vi "FGV test.vi"() -> ()   [LabVIEW 2023]
uses:
  CONTROLS/fgv-status.ctl
panel:
  in  "fgv-status 2":T1
  out "Preis Output 2":dbl
  out "error out":errorcluster
  in  "Preis Input":dbl format="%#_13g"
  in  "error in":errorcluster
  in  "fgv-status":T1
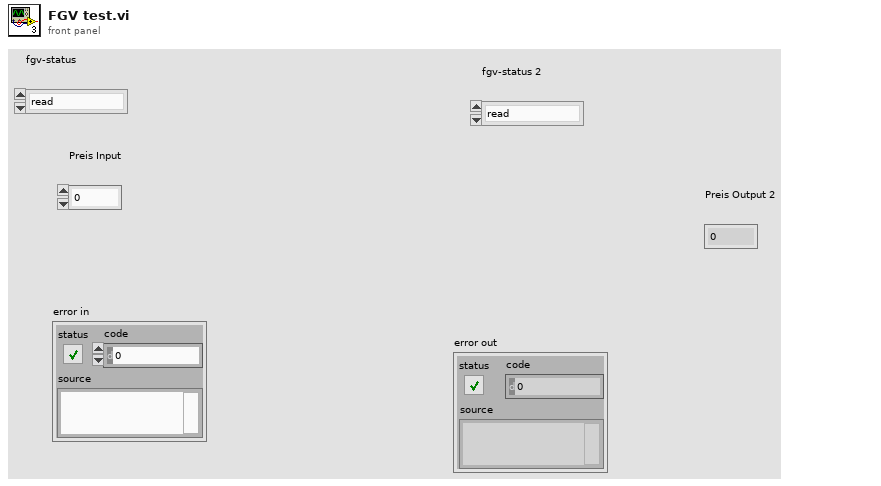
[diagram p1: front panel]
types:
  T1 = typedef "fgv-status.ctl" = enum16{"read", "write"}
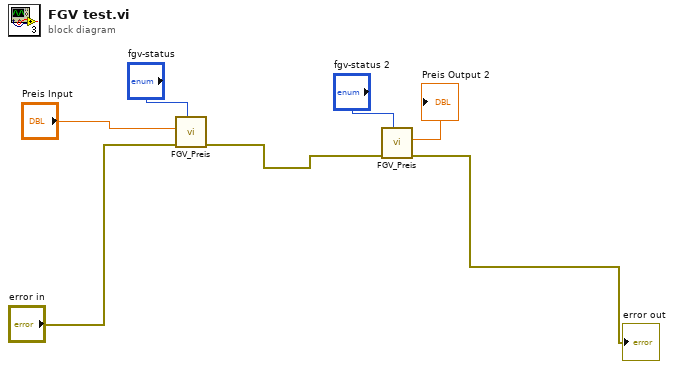
[diagram p0: block diagram]
diagram:
  n1 = call "FGV_Preis.vi"("fgv-status"="fgv-status", "error in"="error in", "Preis Input"="Preis Input") -> ("error out"=w2:errorcluster)  [unwired: 7 in, 1 out]
  n2 = call "FGV_Preis.vi"("fgv-status"="fgv-status 2", "error in"=w2) -> ("error out"=→"error out":errorcluster, "Preis Output"=→"Preis Output 2":dbl)  [unwired: 8 in]
